vi "wireInitializeInput.vi"(8 "error in (no error)":errorcluster, 11 "vi refnum":refnum<vi>) -> (0 "error out":errorcluster, 3 "dup vi refnum":refnum<vi>)   [LabVIEW 2009, in "HGF_VisitorGenerator.lvlib"]
doc: "wire call parent node of visitors init.vi"
uses:
  HGF_VisitorGenerator.lvlib
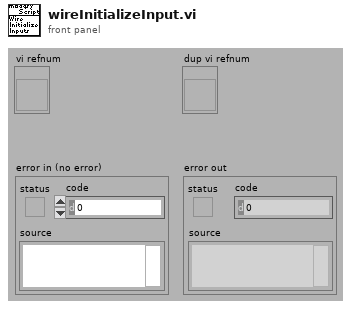
[diagram p1: front panel]
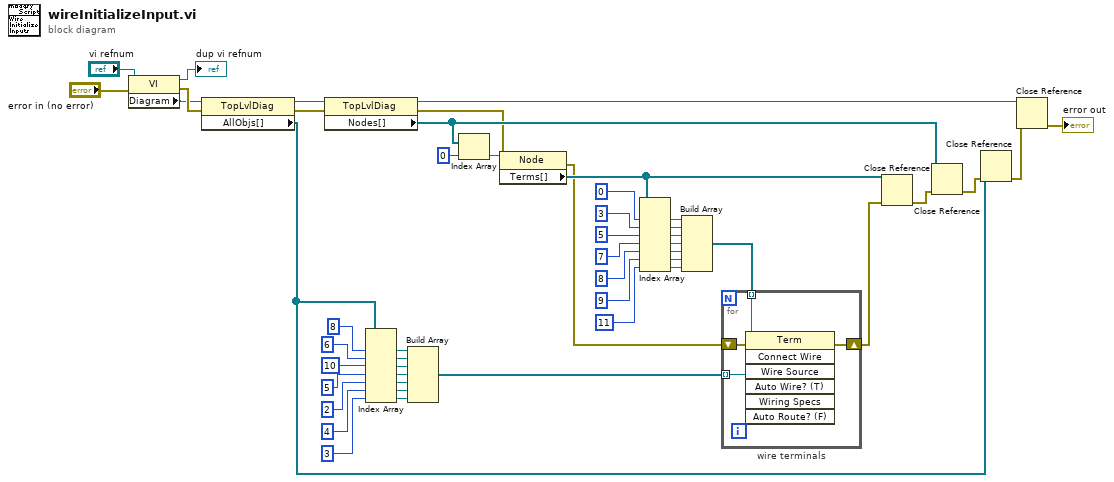
[diagram p0: block diagram]
diagram:
  n1 = property class="VI"(reference="vi refnum", error in="error in (no error)") -> (reference out=→"dup vi refnum":refnum<vi>, error out=w49:errorcluster, "Diagram"=w42:refnum<vi>)
  n2 = property class="TopLvlDiag"(reference=w42, error in=w49) -> (reference out=w41:refnum<vi>, error out=w37:errorcluster, "AllObjs[]"=w27:refnum<vi>[])
  n3 = property class="TopLvlDiag"(reference=w41, error in=w37) -> (reference out=w43:refnum<vi>, error out=w36:errorcluster, "Nodes[]"=w47:refnum<vi>[])
  n4 = Index Array(array=w27, index #1=8 ("index"), index #2=6 ("index"), index #3=10 ("index"), index #4=5 ("index"), index #5=2 ("index"), index #6=4 ("index"), index #7=3 ("index")) -> (element #1=w30:refnum<vi>, element #2=w23:refnum<vi>, element #3=w20:refnum<vi>, element #4=w16:refnum<vi>, element #5=w12:refnum<vi>, element #6=w8:refnum<vi>, element #7=w4:refnum<vi>)
  n5 = Build Array(w30, w23, w20, w16, w12, w8, w4) -> (w29:refnum<vi>[])
  n6 = Index Array(array=w47, index=0) -> (element=w45:refnum<vi>)
  n7 = property class="Node"(reference=w45, error in=w36) -> (error out=w28:errorcluster, "Terms[]"=w34:refnum<vi>[])  [unwired: 1 out]
  n8 = Index Array(array=w34, index #1=0 ("index"), index #2=3 ("index"), index #3=5 ("index"), index #4=7 ("index"), index #5=8 ("index"), index #6=9 ("index"), index #7=11 ("index")) -> (element #1=w35:refnum<vi>, element #2=w24:refnum<vi>, element #3=w21:refnum<vi>, element #4=w18:refnum<vi>, element #5=w14:refnum<vi>, element #6=w10:refnum<vi>, element #7=w6:refnum<vi>)
  n9 = Build Array(w35, w24, w21, w18, w14, w10, w6) -> (w32:refnum<vi>[])
  n10 = for "wire terminals" {
    tunnel: w32 -> [w54] mode=indexing
    tunnel: w29 -> [w51] mode=indexing
    shift-right: [w52] -> w2
    shift-left: w28 -> [w53]
    n11 = invoke class="Term" method="Connect Wire"(reference=w54, error in=w53, "Wire Source"=w51) -> (error out=w52:errorcluster)  [unwired: 4 in, 6 out]
  }
  n12 = Close Reference(reference=w34, error in (no error)=w2) -> (error out=w44:errorcluster)
  n13 = Close Reference(reference=w47, error in (no error)=w44) -> (error out=w39:errorcluster)
  n14 = Close Reference(reference=w27, error in (no error)=w39) -> (error out=w38:errorcluster)
  n15 = Close Reference(reference=w43, error in (no error)=w38) -> (error out=→"error out":errorcluster)
